vi "FGV Klima Option.vi"(6 "Aktion":T1, 9 "PNS vorhanden":u16, 10 "Container":u16, 11 "Klima vorhanden":u16) -> (1 "PNS vorhanden":bool, 2 "Container AMC":bool, 3 "Klimaanlage vorhanden":bool)   [LabVIEW 2020, in "Allgemein.lvlib"]
uses:
  Allgemein.lvlib
  Aktion FGV Klima.ctl
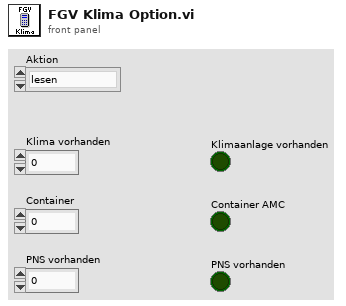
[diagram p1: front panel]
types:
  T1 = typedef "Allgemein.lvlib/Aktion FGV Klima.ctl" = enum16{"lesen", "Klimaanlage", "Container", "PNS"}
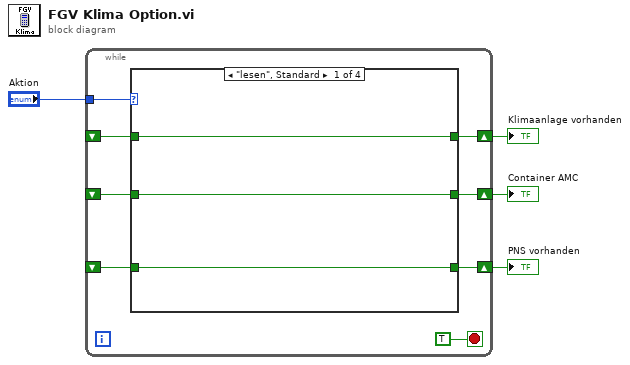
[diagram p0: block diagram]
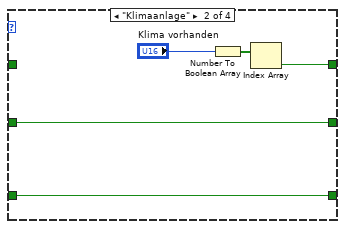
[diagram p2: hidden frame]
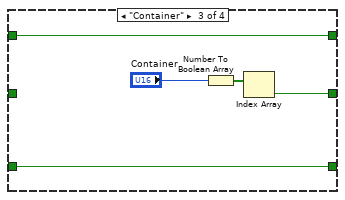
[diagram p3: hidden frame]
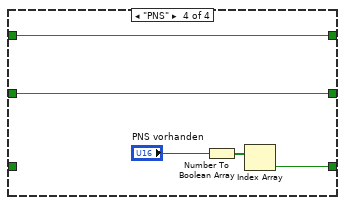
[diagram p4: hidden frame]
diagram:
  n1 = while {
    tunnel: "Aktion" -> [w11]
    shift-right: [w10] -> w3
    shift-left: _ -> [w9]
    shift-right: [w8] -> w2
    shift-left: _ -> [w7]
    shift-right: [w6] -> w1
    shift-left: _ -> [w5]
    stop <- TRUE stop-if-true
    n2 = case shown="\"lesen\", Standard" w11 {
      tunnel: [w15 w18 w23 w28] -> w10
      tunnel: w9 -> [w15 _ w23 w28]
      tunnel: [w14 w17 w22 w26] -> w8
      tunnel: w7 -> [w14 w17 _ w26]
      tunnel: [w13 w16 w21 w27] -> w6
      tunnel: w5 -> [w13 w16 w21 _]
      frame "lesen", Default {
      }
      frame "Klimaanlage" {
        n3 = Number To Boolean Array(number="Klima vorhanden") -> (Boolean array=w19:bool[])
        n4 = Index Array(array=w19) -> (element=w18:bool)  [unwired: 1 in]
      }
      frame "Container" {
        n5 = Number To Boolean Array(number="Container") -> (Boolean array=w24:bool[])
        n6 = Index Array(array=w24) -> (element=w22:bool)  [unwired: 1 in]
      }
      frame "PNS" {
        n7 = Number To Boolean Array(number="PNS vorhanden") -> (Boolean array=w29:bool[])
        n8 = Index Array(array=w29) -> (element=w27:bool)  [unwired: 1 in]
      }
    }
  }
  "Klimaanlage vorhanden" <- w3
  "Container AMC" <- w2
  "PNS vorhanden" <- w1
